vi "InitStringValuesFromRegistry(SubVI).vi"(4 "error in":errorcluster, 5 "String References":refnum<vi>[](array[refnum]), 6 "subkey":string, 7 "root key (HKEY_LOCAL_MACHINE)":T1) -> (0 "error out":errorcluster, 2 "Key Values":string[](array[string]), 3 "Control Labels":string[](array[string]))   [LabVIEW 2015]
uses:
  <vilib>/registry/registry.llb/Registry RtKey.ctl
  <vilib>/registry/registry.llb/Registry SAM.ctl
  <vilib>/registry/registry.llb/Read Registry Value Simple STR.vi
panel:
  out "String Values":string[](array[string])
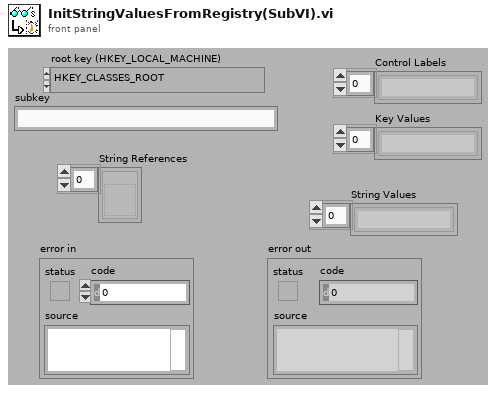
[diagram p1: front panel]
types:
  T1 = typedef "Registry RtKey.ctl" = enum32{"HKEY_CLASSES_ROOT", "HKEY_CURRENT_USER", "HKEY_LOCAL_MACHINE", "HKEY_USERS", "HKEY_PERFORMANCE_DATA", "HKEY_CURRENT_CONFIG", "HKEY_DYN_DATA"}
  T2 = typedef "Registry SAM.ctl" = enum32{"KEY_QUERY_VALUE", "KEY_SET_VALUE", "KEY_CREATE_SUB_KEY", "KEY_ENUMERATE_SUB_KEYS", "KEY_NOTIFY", "KEY_CREATE_LINK", "KEY_READ", "KEY_WRITE", "KEY_ALL_ACCESS", "KEY_READ | KEY_WRITE"}
  T3 = typedef "Registry refnum.ctl" = refnum<k1>
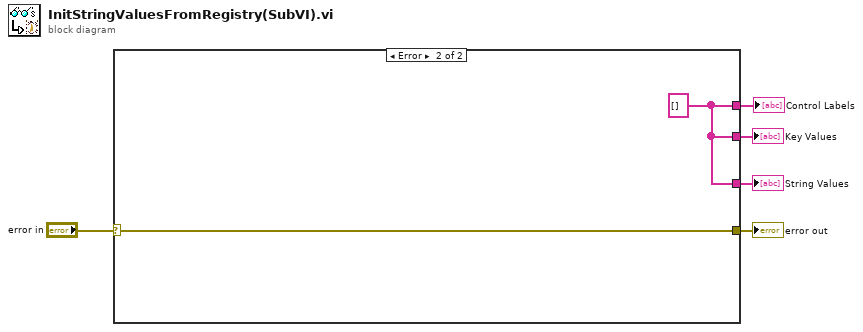
[diagram p0: block diagram]
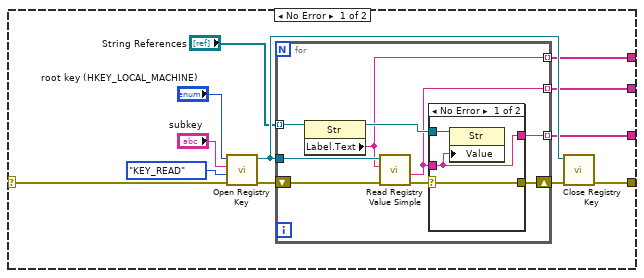
[diagram p2: hidden frame]
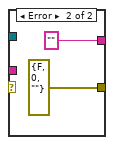
[diagram p3: hidden frame]
diagram:
  n1 = case shown="Error" "error in" {
    selector: "error in" -> [w6 w32]
    tunnel: [w10 w32] -> w4
    tunnel: [w9 w33] -> w3
    tunnel: [w8 w33] -> w2
    tunnel: [w7 w33] -> w1
    frame No Error {
      n2 = call <vilib>:"Open Registry Key.vi"("error in (no error)"=w6, "security access mask (KEY_READ | KEY_WRITE)"=Registry_SAM."KEY_READ", "subkey"="subkey", "root key (HKEY_LOCAL_MACHINE)"="root key (HKEY_LOCAL_MACHINE)") -> ("error out"=w15:errorcluster, "refnum out"=w16:T3)  [unwired: 6 out]
      n3 = for {
        tunnel: "String References" -> [w25] mode=indexing
        shift-right: [w21] -> w17
        shift-left: w15 -> [w24]
        tunnel: w16 -> [w23]
        tunnel: [w20] -> w9 mode=indexing
        tunnel: [w19] -> w8 mode=indexing
        tunnel: [w18] -> w7 mode=indexing
        n4 = property class="Str"(reference=w25) -> (reference out=w26:refnum<vi>, "Label.Text"=w20:string)  [unwired: 1 in, 1 out]
        n5 = call-poly <vilib>:"Read Registry Value Simple.vi"("error in (no error)"=w24, "value"=w20, "refnum"=w23) -> ("error out"=w22:errorcluster, "String/Binary data"=w19:string)  [unwired: 1 in, 4 out]
        n6 = case shown="No Error" w22 {
          selector: w22 -> [w28 _]
          tunnel: w26 -> [w29 _]
          tunnel: w19 -> [w27 _]
          tunnel: [w28 errorcluster {"status"=FALSE, "code"=0, "source"=""} ("error IO")] -> w21
          tunnel: [w27 "" ("String/Binary data")] -> w18
          frame No Error {
            n7 = property class="Str"(reference=w29, "Value"=w27) -> ()  [unwired: 1 in, 2 out]
          }
          frame Error {
          }
        }
      }
      n8 = call <vilib>:"Close Registry Key.vi"("error in (no error)"=w17, "refnum"=w16) -> ("error out"=w10:errorcluster)  [unwired: 5 out]
    }
    frame Error {
      w33 = string[] []
    }
  }
  "error out" <- w4
  "Control Labels" <- w3
  "Key Values" <- w2
  "String Values" <- w1
